vi "Init.vi"(8 "error in (no error)":errorcluster, 11 "Sabritas Actor in":refnum<class "Sabritas Actor.lvclass">) -> (0 "error out":errorcluster, 3 "Sabritas Actor out":refnum<class "Sabritas Actor.lvclass">)   [LabVIEW 2020, in "Sabritas Actor.lvlib" / "Sabritas Actor.lvclass"]
uses:
  Sabritas Actor.lvclass
  Sabritas Actor.lvclass/Sabritas Actor.ctl
  <vilib>/Utility/config.llb/Read Key (Double).vi
  <vilib>/Utility/config.llb/Read Key (String).vi
  <vilib>/Utility/config.llb/NI_LVConfig.lvlib
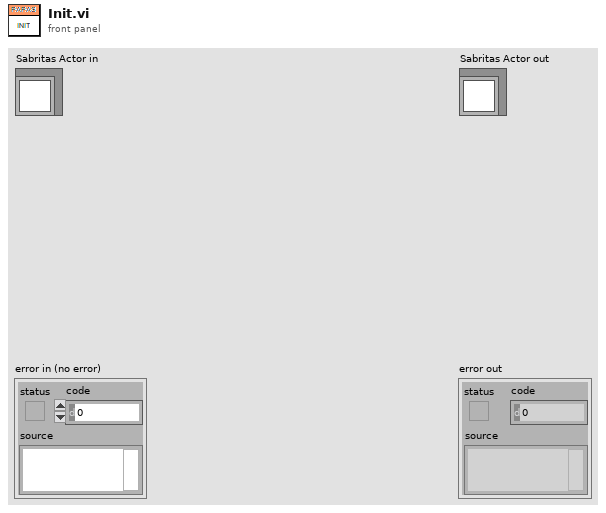
[diagram p1: front panel]
types:
  T1 = typedef "NI_LVConfig.lvlib/Config Data RefNum.ctl" = refnum<k1>
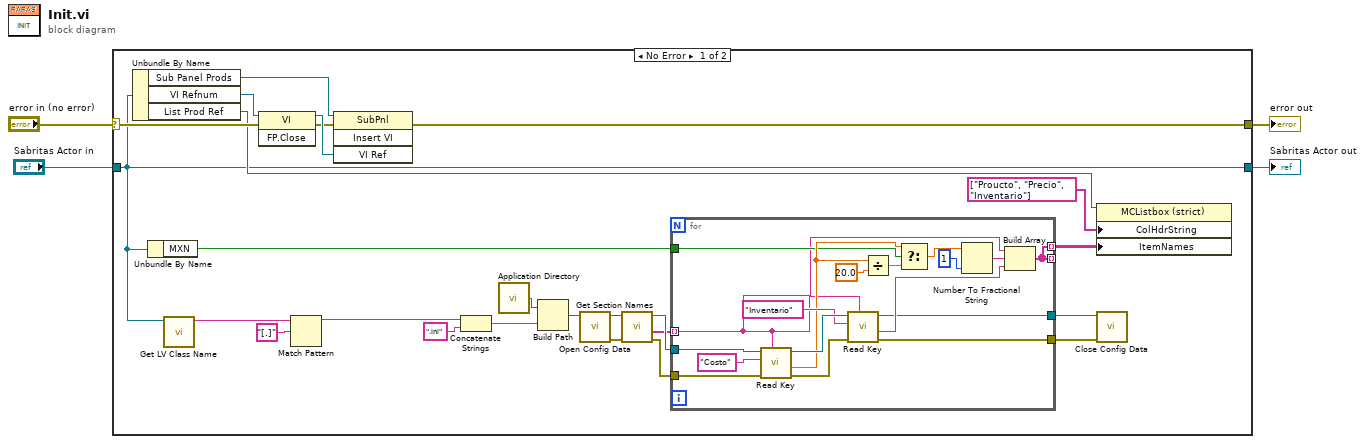
[diagram p0: block diagram]
diagram:
  n1 = case shown="No Error" "error in (no error)" {
    selector: "error in (no error)" -> [w25 w49]
    tunnel: [w26 w49] -> w3
    tunnel: [w5 w48] -> w1
    tunnel: "Sabritas Actor in" -> [w5 w48]
    frame No Error {
      n2 = Unbundle By Name(w5) -> ("Sub Panel Prods"=w28:refnum<vi>, "VI Refnum"=w29:refnum<vi>, "List Prod Ref"=w23:refnum<vi>)
      n3 = Unbundle By Name(w5) -> ("MXN"=w9:bool)
      n4 = call <vilib>:"Get LV Class Name.vi"("object"=w5) -> ("class name"=w13:string)  [unwired: 9 in, 1 out]
      n5 = invoke class="VI" method="FP.Close"(reference=w29, error in=w25) -> (reference out=w27:refnum<vi>, error out=w24:errorcluster)  [unwired: 1 in, 1 out]
      n6 = Match Pattern(string=w13, regular expression="[.]") -> (before substring=w12:string)  [unwired: 1 in, 3 out]
      n7 = invoke class="SubPnl" method="Insert VI"(reference=w28, error in=w24, "VI Ref"=w27) -> (error out=w26:errorcluster)  [unwired: 1 in, 3 out]
      n8 = Concatenate Strings(w12, ".ini" ("string")) -> (w17:string)
      n9 = call <vilib>:"Application Directory.vi"() -> ("Application Directory"=w18:path)
      n10 = Build Path(base path=w18, name or relative path=w17) -> (appended path=w15:path)
      n11 = call <vilib>:"Open Config Data.vi"("configuration file path"=w15) -> ("error out"=w14:errorcluster, "refnum"=w10:T1)  [unwired: 8 in, 1 out]
      n12 = call <vilib>:"Get Section Names.vi"("error in (no error)"=w14, "refnum"=w10) -> ("error out"=w6:errorcluster, "section names"=w7:string[], "refnum out"=w8:T1)  [unwired: 7 in]
      n13 = for {
        tunnel: [w36] -> _ mode=indexing
        tunnel: [w36] -> w22 mode=indexing
        tunnel: [w35] -> w20
        tunnel: [w34] -> w19
        tunnel: w9 -> [w33]
        tunnel: w8 -> [w32]
        tunnel: w7 -> [w31] mode=indexing
        tunnel: w6 -> [w30]
        n14 = call-poly <vilib>:"Read Key.vi"("section"=w31, "error in (no error)"=w30, "key"="Costo", "refnum"=w32) -> ("error out"=w46:errorcluster, "value"=w39:dbl, "refnum out"=w47:T1)  [unwired: 4 in, 1 out]
        n15 = call-poly <vilib>:"Read Key.vi"("section"=w31, "error in (no error)"=w46, "key"="Inventario", "refnum"=w47) -> ("error out"=w35:errorcluster, "value"=w43:string, "refnum out"=w34:T1)  [unwired: 4 in, 1 out]
        n16 = Divide(x=w39, y=20.0) -> (x/y=w37:dbl)
        n17 = Select(t=w39, s=w33, f=w37) -> (s? t:f=w40:dbl)
        n18 = Number To Fractional String(number=w40, precision (6)=i16 1) -> (F-format string=w41:string)  [unwired: 2 in]
        n19 = Build Array(w31, w41, w43) -> (w36:string[])
      }
      n20 = property class="MCListbox (strict)"(reference=w23, "ColHdrString"=string[] ["Proucto", "Precio", "Inventario"] ("Column Header Strings[]"), "ItemNames"=w22) -> ()  [unwired: 1 in, 2 out]
      n21 = call <vilib>:"Close Config Data.vi"("error in (no error)"=w20, "refnum"=w19) -> ()  [unwired: 8 in, 2 out]
    }
    frame Error {
    }
  }
  "error out" <- w3
  "Sabritas Actor out" <- w1
